vi "Multi-Loop Humidity Control.vi"(5 "Use Tair":bool, 6 "dt (s)":dbl=2.0, 7 "PID":T1(array[cluster]) {"derivative time (Td, min)" format="%.3f"; "integral time (Ti, min)" format="%.3f"; "proportional gain (Kc)" format="%.3f"}, 8 "error in":errorcluster, 9 "Tair":dbl[](array[numeric]) format="%#.2g", 10 "RH meas":dbl[](array[numeric]) format="%.2f", 11 "RHsp":dbl[](array[numeric]) format="%.2f") -> (0 "error out":errorcluster, 2 "PID Out":dbl[](array[numeric]) format="%.2f", 3 "Td (degC)":dbl[](array[numeric]) format="%.2f")   [LabVIEW 2013]
doc: "This VI updates the temperature setpoint on the UHSAS RH control system using a PID algorithm. For this algortihm:\n* The error, e, is RHsp - RHmeas\n* The output of the control loop is u. This variable is transformed to temperature by associating it with an assumed saturator efficieny. Ideally, the saturator efficiency is 1, but there may be uncertainties that limit this. There fore, the output u, is transformed to an efficiency k by using the following assumptions:\n * when RHmeas < RHsp, k <1\n * when RHmeas > RHsp, k >1\n * when RHmeas = RHsp, k = 1\n To relate temperature to this k, we assume that the k*RHcal= k*esat(Tsp)/esat(Tair)=RHmeas. From this equation, we can calculate the dewpoint of the air exiting the saturator based on the efficiency term k \n* The dewpoint calculated above is the new saturator setpoint."
uses:
  <vilib>/addons/control/pid/pid.llb/PID (DBL Array).vi
  <vilib>/addons/control/pid/pid.llb/PID Percentage to EGU (DBL Array).vi
  <vilib>/addons/control/pid/NI_PID_pid.lvlib
  General/Atmospheric/Atmospheric Library.lvlib
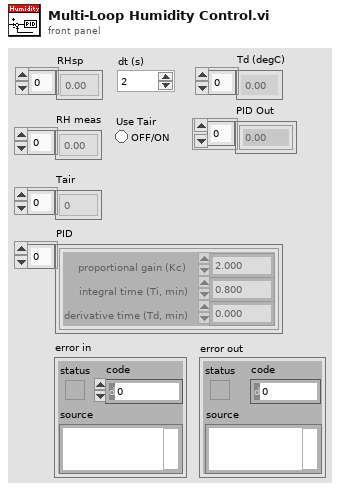
[diagram p1: front panel]
types:
  T1 = cluster{"proportional gain (Kc)":dbl, "integral time (Ti, min)":dbl, "derivative time (Td, min)":dbl}[]
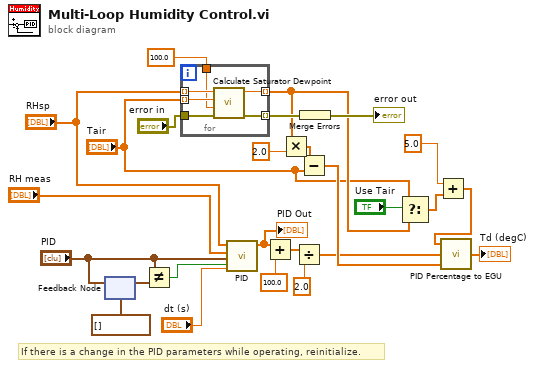
[diagram p0: block diagram]
diagram:
  # "If there is a change in the PID parameters while operating, reinitialize."
  n1 = feedback-in #1("PID") -> ()
  n2 = feedback #1(T1 []) -> (w24:T1)
  n3 = Not Equal?(x="PID", y=w24) -> (x != y?=w23:bool)
  n4 = for {
    tunnel: "error in" -> [w32]
    tunnel: [w31] -> w14 mode=indexing
    tunnel: [w30] -> w5 mode=indexing
    tunnel: "RHsp" -> [w29] mode=indexing
    tunnel: "Tair" -> [w28] mode=indexing
    tunnel: 100.0 ("RH_sat_out") -> [w27]
    n5 = call "Calculate Saturator Dewpoint.vi"("error in"=w32, "RH_sat_out"=w27, "Tair"=w28, "RH_tar"=w29) -> ("error out"=w31:errorcluster, "Td"=w30:dbl)  [unwired: 6 in]
  }
  n6 = call-poly <vilib>:"PID.vi"("reinitialize? (F)"=w23, "dt (s)"="dt (s)", "PID gains"="PID", "process variable"="RH meas", "setpoint"="RHsp") -> ("output"=w20:dbl[])  [unwired: 5 in, 1 out]
  "PID Out" <- w20
  n7 = Add(x=w20, y=100.0) -> (x+y=w18:dbl[])
  n8 = Multiply(x=w5, y=2.0) -> (x*y=w21:dbl[])
  n9 = Divide(x=w18, y=2.0) -> (x/y=w15:dbl[])
  n10 = Subtract(x=w21, y="Tair") -> (x-y=w16:dbl[])
  n11 = Merge Errors(w14) -> (→"error out":errorcluster)
  n12 = Select(t="Tair", s="Use Tair", f=w5) -> (s? t:f=w3:dbl[])
  n13 = Add(x=5.0, y=w3) -> (x+y=w1:dbl[])
  n14 = call-poly <vilib>:"PID Percentage to EGU.vi"("minimum (EGU)"=w16, "% span"=w15, "maximum (EGU)"=w1) -> ("output (EGU)"=→"Td (degC)":dbl[])  [unwired: 1 in]
